vi "Base-Software.vi"(8 "error in":errorcluster, 11 "Launcher in":refnum<class "Launcher.lvclass">) -> (0 "error out":errorcluster, 3 "Launcher out":refnum<class "Launcher.lvclass">)   [LabVIEW 2019, in "Launcher.lvlib" / "Launcher.lvclass"]
uses:
  Library/Launcher.lvclass
  Library/Launcher.lvclass/Launcher.ctl
  builds/Base Software/Base Software.lvlibp/Project/Base Software.lvclass
panel:
  out "Application Name":string
  out "Current Action":string caption="Current Action:"
  out "Waiting Lights":T1
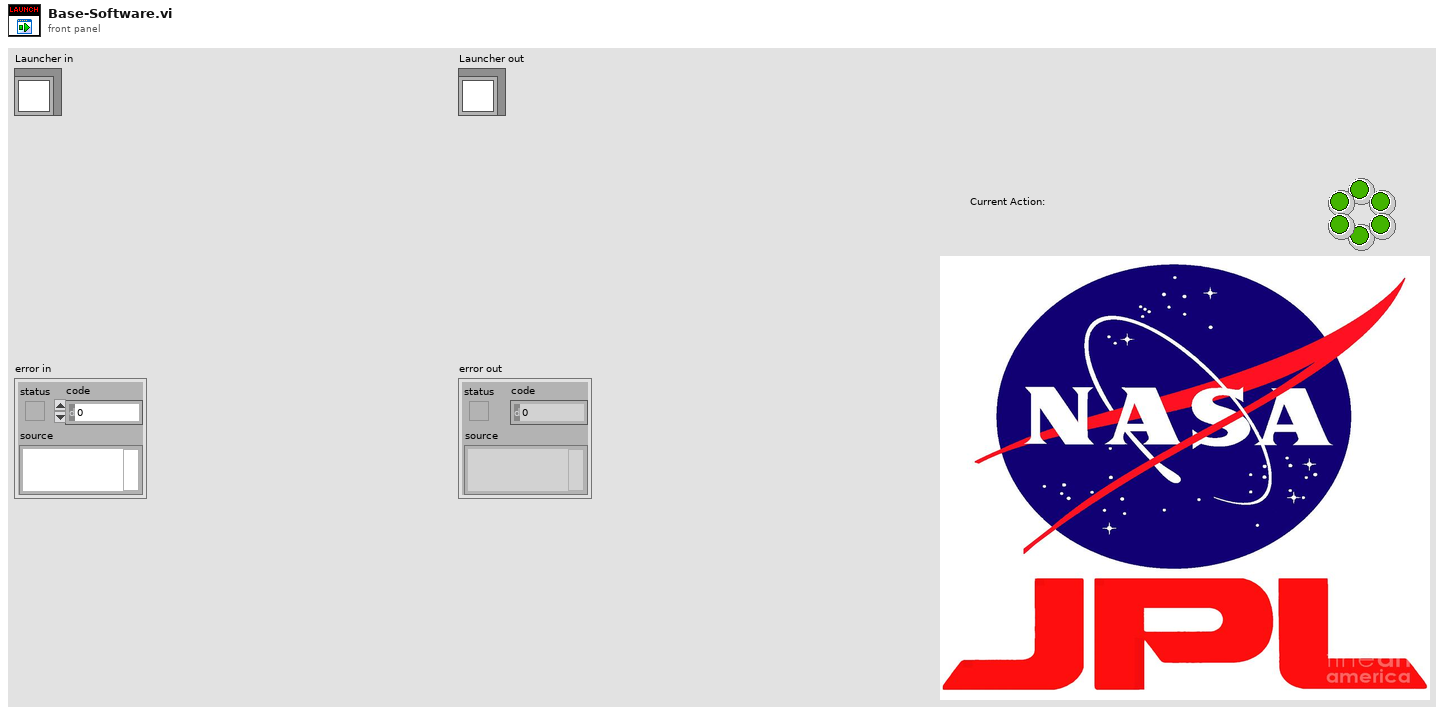
[diagram p1: front panel]
types:
  T1 = cluster{"wait 1":bool, "wait 2":bool, "wait 3":bool, "wait 4":bool, "wait 5":bool, "wait 6":bool}
  T2 = enum32{"Invalid", "Standard", "Closed", "Hidden", "Minimized", "Maximized"}
  T3 = cluster{"[0]":bool, "[1]":bool, "[2]":bool, "[3]":bool, "[4]":bool, "[5]":bool}
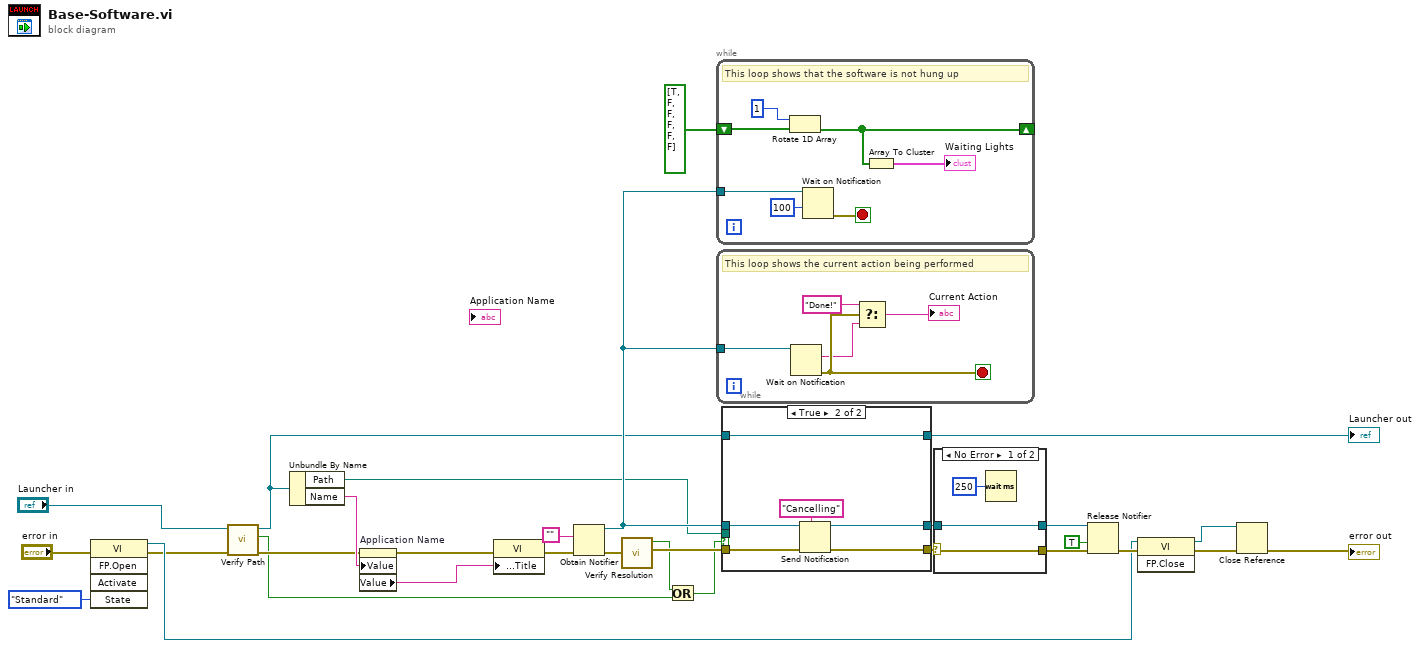
[diagram p0: block diagram]
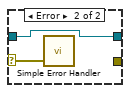
[diagram p2: hidden frame]
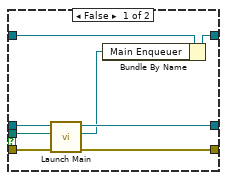
[diagram p3: hidden frame]
diagram:
  n1 = invoke class="VI" method="FP.Open"(error in="error in", "State"=T2."Standard") -> (reference out=w14:refnum<vi>, error out=w6:errorcluster)  [unwired: 3 in, 3 out]
  n2 = call "Verify Path.vi"("error in"=w6, "Launcher in"="Launcher in") -> ("error out"=w5:errorcluster, "Abort?"=w2:bool, "Launcher out"=w4:refnum<class "Launcher.lvclass">)  [unwired: 7 in]
  n3 = Unbundle By Name(w4) -> ("Path"=w8:path, "Name"=w11:string)
  n4 = property on="Application Name" class="Str"(error in=w5, "Value"=w11) -> (error out=w12:errorcluster, "Value"=w10:string)  [unwired: 1 in, 1 out]
  n5 = property class="VI"(error in=w12, "Front Panel.Title"=w10) -> (error out=w28:errorcluster)  [unwired: 1 in, 1 out]
  n6 = Obtain Notifier(notification data type="", error in (no error)=w28) -> (notifier out=w25:refnum<notifier>, error out=w27:errorcluster)  [unwired: 2 in, 1 out]
  n7 = call "Verify Resolution.vi"("error in"=w27) -> ("error out"=w26:errorcluster, "Abort Launch"=w3:bool)  [unwired: 9 in]
  n8 = Or(x=w3, y=w2) -> (x .or. y?=w1:bool)
  n9 = while {
    tunnel: w25 -> [w36]
    shift-right: [w32] -> _
    shift-left: bool[] [TRUE, FALSE, FALSE, FALSE, FALSE, FALSE] -> [w34]
    stop <- w33 stop-if-true
    # "This loop shows that the software is not hung up"
    n10 = Rotate 1D Array(1:w34, 2:1 ("n")) -> (0:w32:bool[])
    n11 = Wait on Notification(notifier=w36, timeout in ms (-1)=100) -> (error out=w33:errorcluster)  [unwired: 2 in, 3 out]
    n12 = Array To Cluster(array=w32) -> (cluster=→"Waiting Lights":T3)
  }
  n13 = while {
    tunnel: w25 -> [w42]
    stop <- w41 stop-if-true
    # "This loop shows the current action being performed"
    n14 = Wait on Notification(notifier=w42) -> (notification=w40:string, error out=w41:errorcluster)  [unwired: 3 in, 2 out]
    n15 = Select(t="Done!", s=w41, f=w40) -> (s? t:f=→"Current Action":string)
  }
  n16 = case shown="True" w1 {
    tunnel: w26 -> [w48 w56]
    tunnel: w25 -> [w50 w55]
    tunnel: [w47 w52] -> w24
    tunnel: [w46 w53] -> w23
    tunnel: w8 -> [w49 _]
    tunnel: w4 -> [w45 w51]
    tunnel: [w44 w51] -> w9
    frame False {
      n17 = call "Launch Main.vi"("error in"=w48, "Path"=w49, "Notifier in"=w50) -> ("error out"=w47:errorcluster, "Main Enqueuer"=w43:refnum<class "Message Enqueuer.lvclass">, "Notifier out"=w46:refnum<notifier>)  [unwired: 6 in]
      n18 = Bundle By Name(cluster=w45, "Main Enqueuer"=w43) -> (w44:refnum<class "Launcher.lvclass">)
    }
    frame True {
      n19 = Send Notification(notification="Cancelling", notifier=w55, error in (no error)=w56) -> (notifier out=w53:refnum<notifier>, error out=w52:errorcluster)
    }
  }
  "Launcher out" <- w9
  n20 = case shown="No Error" w24 {
    tunnel: [w58 _] -> w22
    selector: w24 -> [w58 w61]
    tunnel: w23 -> [w57 w60]
    tunnel: [w57 w60] -> w21
    frame No Error {
      n21 = Wait (ms)(milliseconds to wait=u32 250) -> ()  [unwired: 1 out]
    }
    frame Error {
      n22 = call <vilib>:"Simple Error Handler.vi"("error in (no error)"=w61) -> ()  [unwired: 4 in, 5 out]
    }
  }
  n23 = Release Notifier(notifier=w21, force destroy? (F)=TRUE, error in (no error)=w22) -> (error out=w18:errorcluster)  [unwired: 2 out]
  n24 = invoke class="VI" method="FP.Close"(reference=w14, error in=w18) -> (reference out=w19:refnum<vi>, error out=w20:errorcluster)  [unwired: 1 in, 1 out]
  n25 = Close Reference(reference=w19, error in (no error)=w20) -> (error out=→"error out":errorcluster)
